vi "RFmx LUT Apply DPD.vi"(0 "RFmx Instrument Handle In":refnum<k21> caption="Instrument Handle In", 1 "Selector String":string, 5 "SG instrument handle":refnum<k15>, 7 "RFmx LUT Configuration":T4={"Threshold Enabled"=1, "Threshold Type"=0, "Threshold Level (dB or dBm)"=-20.0, "LUT Step Size (dB)"=0.1, "LUT Correction Type"=0, " LUT Type"=0} {"LUT Type" items=["Log", "Linear"]; "LUT Correction Type" items=["Magnitude and Phase", "Magnitude Only", "Phase Only"]; "Threshold Level (dB or dBm)" format="%.2g"; "Threshold Type" items=["Relative", "Absolute"]; "Threshold Enabled" items=["False", "True"]}, 9 "RFmx DPD Common Configuration":T1={"DPD Measurement Interval (s)"=0.0001, "Sample Rate Mode"=1, "Sample Rate (S/s)"=120000000.0, "Signal Type"=0, "Pre DPD CFR Enabled"=0, "Apply DPD CFR Enabled"=0, "DUT Average Input Power (dBm)"=-15.0} {"DUT Average Input Power (dBm)" format="%.2f"; "Apply DPD CFR Enabled" items=["False", "True"]; "Pre DPD CFR Enabled" items=["False", "True"]; "Signal Type" items=["Modulated", "Tones"]; "Sample Rate (S/s)" format="%.2p"; "Sample Rate Mode" items=["User", "Reference Waveform"]; "DPD Measurement Interval (s)" format="%#.2p"}, 11 "error in (no error)":errorcluster, 12 "Waveform":T3={"Waveform Name"="Wfm", "Waveform"={"x0"=0.0, "dx"=0.0, "y"=[]}, "Signal Bandwidth (Hz)"=0.0, "PAPR (dB)"=0.0, "Burst Length (s)"=0.0, "Sample Rate"=0.0, "Burst Start Locations"=[], "Burst Stop Locations"=[], "Idle Duration Present?"=FALSE, "Runtime Scaling"=0.0} {"Runtime Scaling" format="%#_6p"; "Sample Rate" format="%#_6p"; "Burst Length (s)" format="%#_6p"; "PAPR (dB)" format="%.2f"; "Signal Bandwidth (Hz)" format="%#_6p"; "Waveform"."y" format="%.2f"; "Waveform"."dx" format="%^.2e"; "Waveform"."x0" format="%^.2e"}) -> (4 "RFmx Instrument Handle Out":refnum<k21> caption="Instrument Handle Out", 6 "SG instrument handle out":refnum<k15>, 8 "RFmx LUT Results":T2={"Waveform Out"={"x0"=0.0, "dx"=0.0, "y"=[]}, "Post DPD PAPR (dB)"=-1.0, "Power Offset (dB)"=-1.0, "Input Powers"=[], "Complex Gains"=[]} {"Power Offset (dB)" format="%.2f"; "Post DPD PAPR (dB)" format="%.2f"; "Waveform Out"."y" format="%.2f"; "Waveform Out"."dx" format="%^.2e"; "Waveform Out"."x0" format="%^.2e"}, 15 "error out":errorcluster)   [LabVIEW 2016, in "DPD.lvlib"]
uses:
  DPD.lvlib
  SG/SG.lvlib
  <vilib>/RFmx/SpecAn/mx/RFmxSpecAn.llb/RFmxSpecAn DPD Fetch Lookup Table.vi
  Typedefs/RFmx LUT Results.ctl
  Typedefs/RFmx LUT Configuration.ctl
  SG/Typedefs/Waveform.ctl
  Typedefs/RFmx DPD Common Configuration.ctl
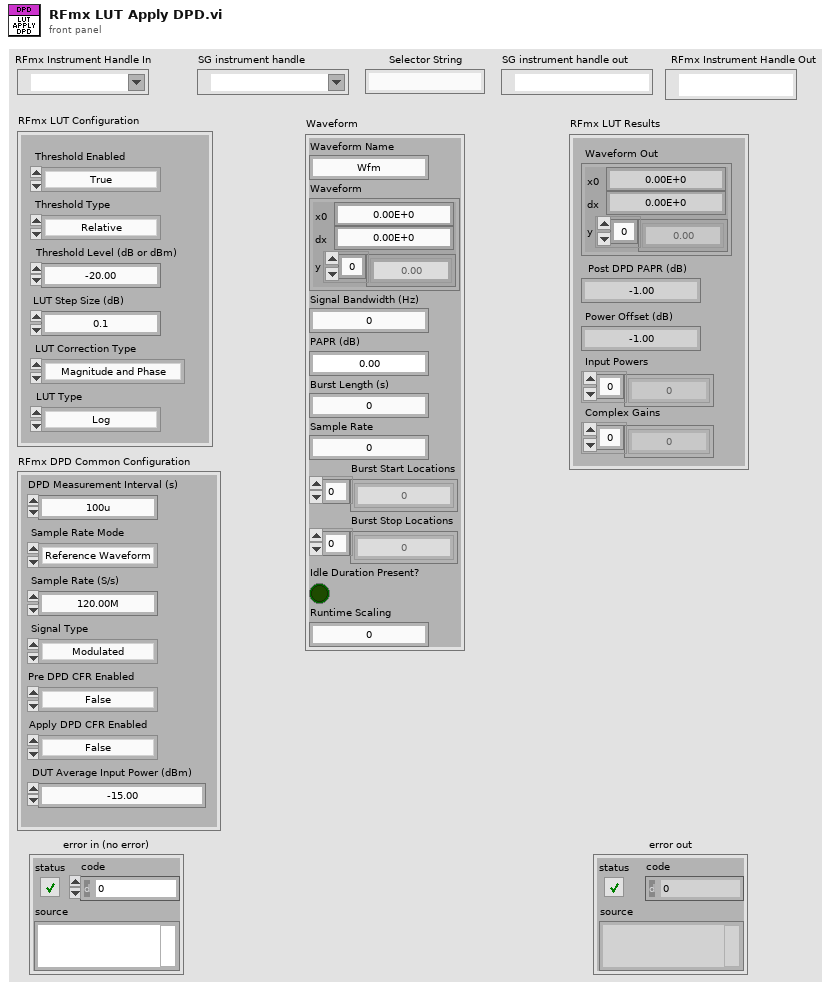
[diagram p1: front panel]
types:
  T1 = typedef "DPD.lvlib/RFmx DPD Common Configuration.ctl" = cluster{"DPD Measurement Interval (s)":dbl, "Sample Rate Mode":i32, "Sample Rate (S/s)":dbl, "Signal Type":i32, "Pre DPD CFR Enabled":i32, "Apply DPD CFR Enabled":i32, "DUT Average Input Power (dBm)":dbl}
  T2 = typedef "DPD.lvlib/RFmx LUT Results.ctl" = cluster{"Waveform Out":cluster{"x0":dbl, "dx":dbl, "y":csg[]}, "Post DPD PAPR (dB)":dbl, "Power Offset (dB)":dbl, "Input Powers":sgl[], "Complex Gains":csg[]}
  T3 = typedef "SG.lvlib/Waveform.ctl" = cluster{"Waveform Name":string, "Waveform":cluster{"x0":dbl, "dx":dbl, "y":csg[]}, "Signal Bandwidth (Hz)":dbl, "PAPR (dB)":dbl, "Burst Length (s)":dbl, "Sample Rate":dbl, "Burst Start Locations":i32[], "Burst Stop Locations":i32[], "Idle Duration Present?":bool, "Runtime Scaling":dbl}
  T4 = typedef "DPD.lvlib/RFmx LUT Configuration.ctl" = cluster{"Threshold Enabled":i32, "Threshold Type":i32, "Threshold Level (dB or dBm)":dbl, "LUT Step Size (dB)":dbl, "LUT Correction Type":i32, " LUT Type":i32}
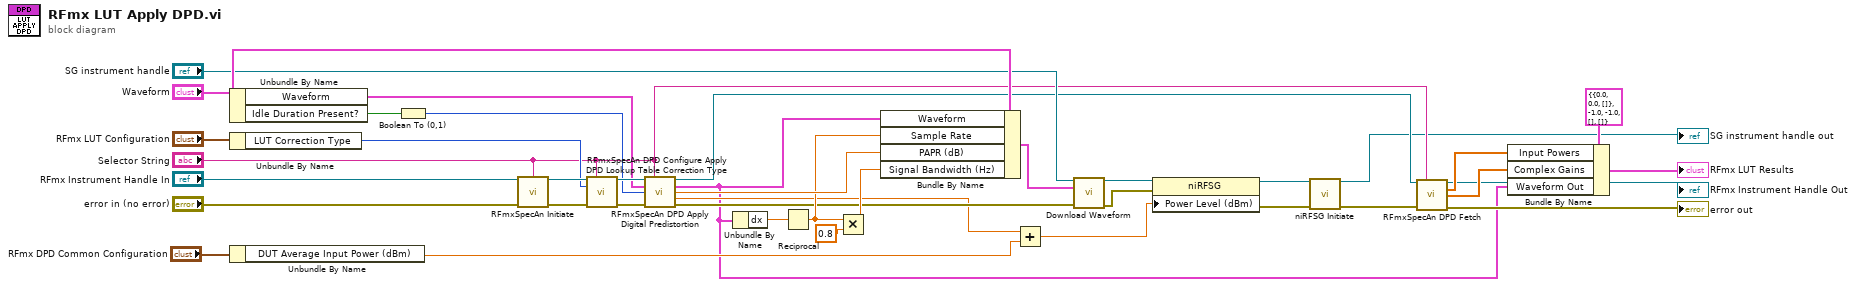
[diagram p0: block diagram]
diagram:
  n1 = Unbundle By Name("Waveform") -> ("Waveform"=w31:cluster{"x0":dbl, "dx":dbl, "y":csg[]}, "Idle Duration Present?"=w30:bool)
  n2 = Unbundle By Name("RFmx LUT Configuration") -> ("LUT Correction Type"=w32:i32)
  n3 = Unbundle By Name("RFmx DPD Common Configuration") -> ("DUT Average Input Power (dBm)"=w18:dbl)
  n4 = Boolean To (0,1)(Boolean=w30) -> (0, 1=w29:i16)
  n5 = call <vilib>:"RFmxSpecAn Initiate.vi"("Instrument Handle In"="RFmx Instrument Handle In", "Result Name"="Selector String", "error in (no error)"="error in (no error)") -> ("Instrument Handle Out"=w38:refnum<k21>, "error out"=w37:errorcluster)  [unwired: 10 in, 1 out]
  n6 = call <vilib>:"RFmxSpecAn DPD Configure Apply DPD Lookup Table Correction Type.vi"("Instrument Handle In"=w38, "Selector String"="Selector String", "LUT Correction Type"=w32, "error in (no error)"=w37) -> ("Instrument Handle Out"=w36:refnum<k21>, "error out"=w35:errorcluster)  [unwired: 10 in]
  n7 = call <vilib>:"RFmxSpecAn DPD Apply Digital Predistortion.vi"("Instrument Handle In"=w36, "Selector String"="Selector String", "Waveform In"=w31, "Idle Duration Present"=w29, "error in (no error)"=w35) -> ("Instrument Handle Out"=w11:refnum<k21>, "Waveform Out"=w4:cluster{"x0":dbl, "dx":dbl, "y":csg[]}, "PAPR (dB)"=w27:dbl, "Power Offset (dB)"=w17:dbl, "error out"=w20:errorcluster)  [unwired: 6 in]
  n8 = Unbundle By Name(w4) -> ("dx"=w26:dbl)
  n9 = Reciprocal(x=w26) -> (1/x=w25:dbl)
  n10 = Multiply(x=w25, y=0.8) -> (x*y=w23:dbl)
  n11 = Bundle By Name(cluster="Waveform", "Waveform"=w4, "Sample Rate"=w25, "PAPR (dB)"=w27, "Signal Bandwidth (Hz)"=w23) -> (w21:T3)
  n12 = Add(x=w17, y=w18) -> (x+y=w14:dbl)
  n13 = call "Download Waveform.vi"("RFSG handle"="SG instrument handle", "Waveform In"=w21, "error in (no error)"=w20) -> ("RFSG handle out"=w16:refnum<k15>, "error out"=w15:errorcluster)  [unwired: 11 in]
  n14 = property class="niRFSG"(reference=w16, error in=w15, "Power Level (dBm)"=w14) -> (reference out=w13:refnum<k15>, error out=w12:errorcluster)
  n15 = call <instrlib>:"niRFSG Initiate.vi"("instrument handle"=w13, "error in"=w12) -> ("instrument handle out"=→"SG instrument handle out":refnum<k15>, "error out"=w10:errorcluster)  [unwired: 12 in]
  n16 = call-poly <vilib>:"RFmxSpecAn DPD Fetch.vi"("Instrument Handle In"=w11, "Selector String"="Selector String", "error in (no error)"=w10) -> ("Instrument Handle Out"=→"RFmx Instrument Handle Out":refnum<k21>, "Input Powers"=w8:sgl[], "Complex Gains"=w7:csg[], "error out"=→"error out":errorcluster)  [unwired: 9 in]
  n17 = Bundle By Name(cluster=T2 {"Waveform Out"={"x0"=0.0, "dx"=0.0, "y"=[]}, "Post DPD PAPR (dB)"=-1.0, "Power Offset (dB)"=-1.0, "Input Powers"=[], "Complex Gains"=[]} ("RFmxLUT Results"), "Input Powers"=w8, "Complex Gains"=w7, "Waveform Out"=w4) -> (→"RFmx LUT Results":T2)
